vi "Calculate Scaling Factors.vi"(8 "Max Picture Size Y":u32=300, 9 "Max Picture Size X":u32=300, 10 "Panel Height":u32, 11 "Panel Width":u32) -> (1 "Scale Factor":dbl, 2 "Picture Y":i32, 3 "Picture X":i32)   [LabVIEW 2018]
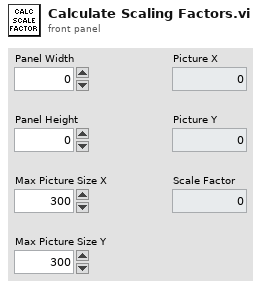
[diagram p1: front panel]
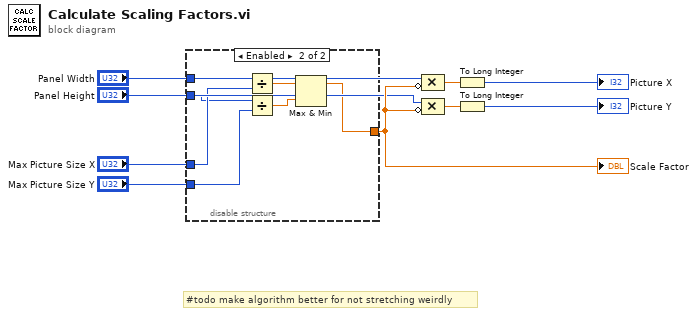
[diagram p0: block diagram]
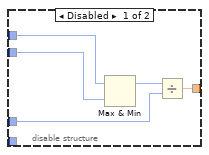
[diagram p2: hidden frame]
diagram:
  # "#todo make algorithm better for not stretching weirdly"
  n1 = disable-structure shown="Enabled" {
    disable-tunnel: [w14 w15] -> w9
    disable-tunnel: "Panel Height" -> [w13 w19]
    disable-tunnel: "Panel Width" -> [w12 w21]
    disable-tunnel: "Max Picture Size X" -> [w11 w20]
    disable-tunnel: "Max Picture Size Y" -> [_ w18]
    frame Disabled {
      n2 = Max & Min(x=w12, y=w13) -> (max(x,y)=w10:u32)  [unwired: 1 out]
      n3 = Divide(x=w10, y=w11) -> (x/y=w14:dbl)
    }
    frame Enabled {
      n4 = Divide(x=w21, y=w20) -> (x/y=w17:dbl)
      n5 = Divide(x=w19, y=w18) -> (x/y=w16:dbl)
      n6 = Max & Min(x=w17, y=w16) -> (max(x,y)=w15:dbl)  [unwired: 1 out]
    }
  }
  "Scale Factor" <- w9
  n7 = Compound Arithmetic op=MULTIPLY("Panel Width", invert w9) -> (w5:dbl)
  n8 = Compound Arithmetic op=MULTIPLY("Panel Height", invert w9) -> (w6:dbl)
  n9 = To Long Integer(number=w5) -> (32bit integer=→"Picture X":i32)
  n10 = To Long Integer(number=w6) -> (32bit integer=→"Picture Y":i32)
